vi "ParseControllerPacket.vi"(8 "error in (no error)":errorcluster, 11 "Hex String":string) -> (0 "error out":errorcluster, 3 "Status":T4, 5 "Parameters":T1)   [LabVIEW 2014]
uses:
  Status.ctl
  Parameters.ctl
  PID Mode.ctl
  InputSimulationMode.ctl
panel:
  out "rest of the binary string":string
  out "Binary String":string
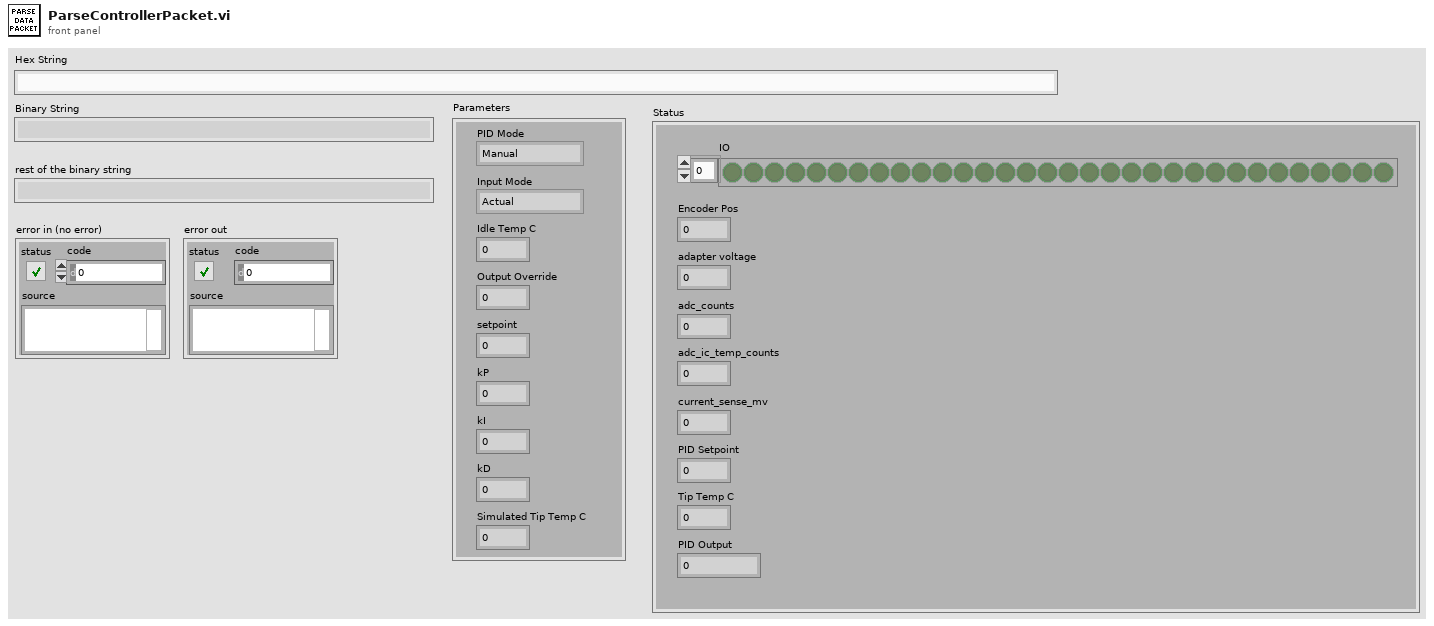
[diagram p1: front panel]
types:
  T1 = typedef "Parameters.ctl" = cluster{"PID Mode":T2, "Input Mode":T3, "Idle Temp C":i16, "Output Override":i16, "setpoint":sgl, "kP":sgl, "kI":sgl, "kD":sgl, "Simulated Tip Temp C":sgl}
  T2 = typedef "PID Mode.ctl" = enum8{"Manual", "Automatic"}
  T3 = typedef "InputSimulationMode.ctl" = enum8{"Actual", "Simulated"}
  T4 = typedef "Status.ctl" = cluster{"IO":bool[], "Encoder Pos":i16, "adapter voltage":i16, "adc_counts":i16, "adc_ic_temp_counts":i16, "current_sense_mv":i16, "PID Setpoint":sgl, "Tip Temp C":sgl, "PID Output":sgl}
  T5 = enum16{"big-endian, network order", "native, host order", "little-endian"}
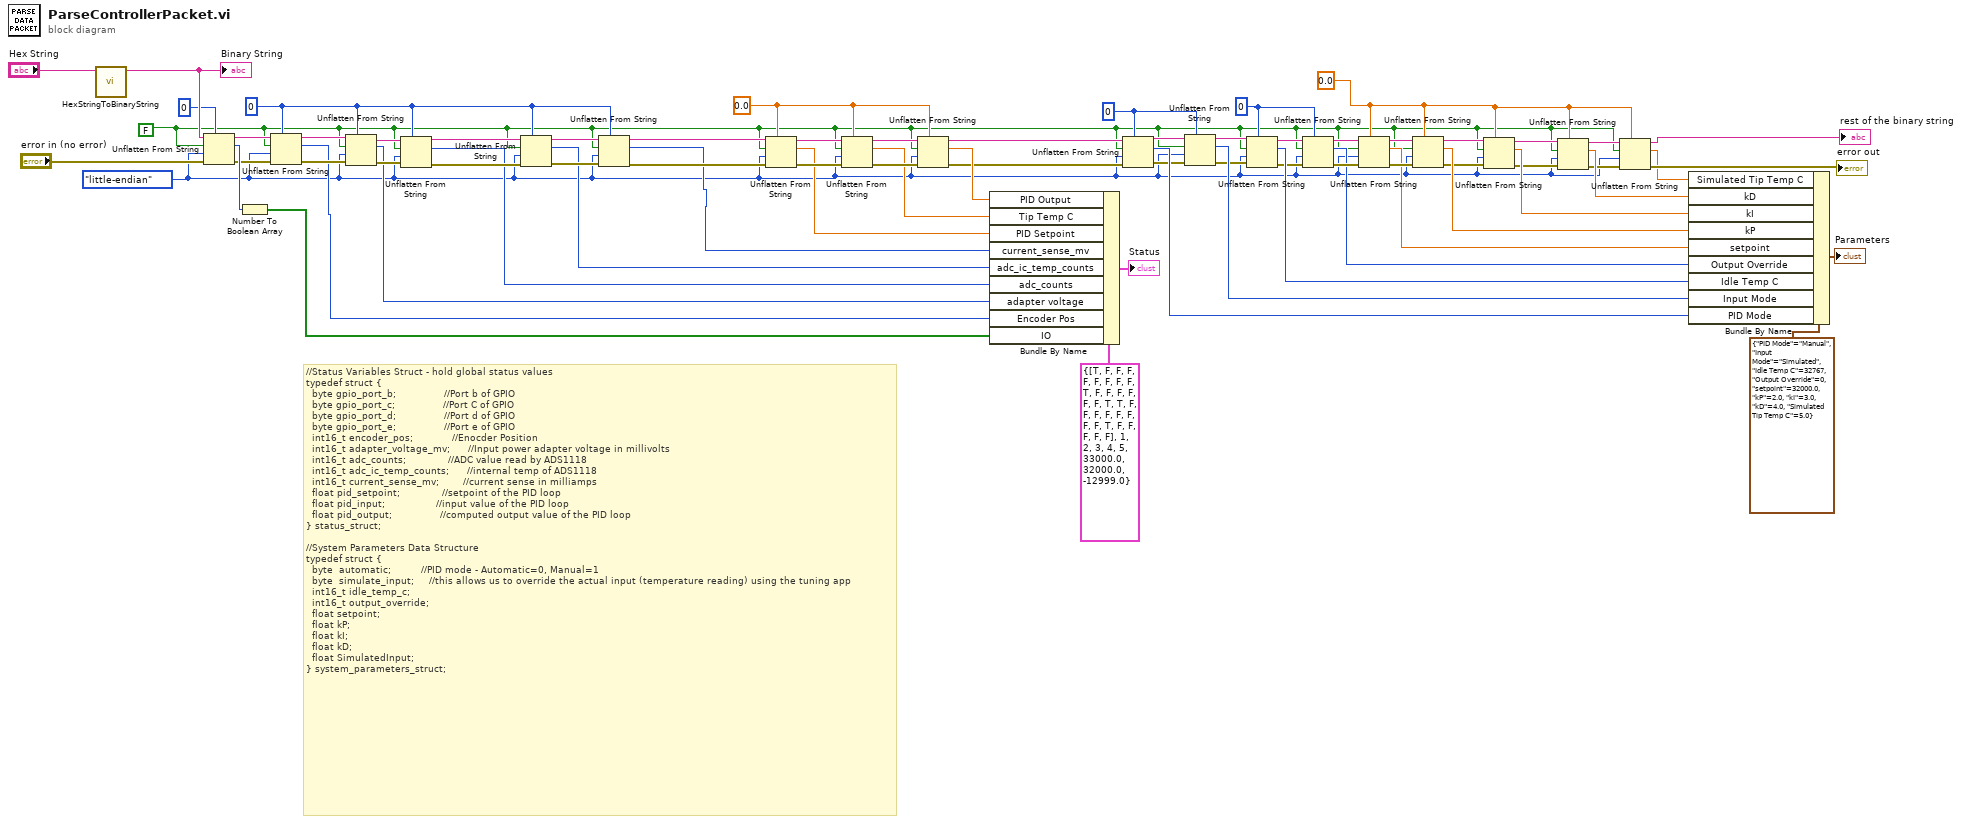
[diagram p0: block diagram]
diagram:
  w4 = sgl 0.0
  w9 = i16 0
  w31 = u8 0
  w49 = sgl 0.0
  w56 = i16 0
  w2 = T5."little-endian" ("byte order (0:big-endian, network order)")
  w3 = FALSE ("data includes array or string size? (T)")
  # "//Status Variables Struct - hold global status values\ntypedef struct {\n  byte gpio_port_b;                //Port b of GPIO\n  byte gpio_port_c;                //Port C of GPIO\n  byte gpio_port_d;                //Port d of GPIO\n  byte gpio_port_e;                //Port e of GPIO\n  int16_t encoder_pos;             //Enocder Position\n  int16_t adapter_voltage_mv;      //Input power adapter voltage in millivolts\n  int16_t adc_counts;              //ADC value read by ADS1118\n  int16_t adc_ic_temp_counts;      //internal temp of ADS1118\n  int16_t current_sense_mv;        //current sense in milliamps\n  float pid_setpoint;              //setpoint of the PID loop\n  float pid_input;                 //input value of the PID loop\n  float pid_output;                //computed output value of the PID loop\n} status_struct;\n\n//System Parameters Data Structure\ntypedef struct {\n  byte  automatic;          //PID mode - Automatic=0, Manual=1\n  byte  simulate_input;     //this allows us to override the actual input (temperature reading) using the tuning app\n  int16_t idle_temp_c;\n  int16_t output_override;\n  float setpoint;\n  float kP;\n  float kI;\n  float kD;\n  float SimulatedInput;\n} system_parameters_struct;"
  n1 = call "HexStringToBinaryString.vi"("Hex String"="Hex String") -> ("Binary String"=w69:string)  [unwired: 10 in]
  "Binary String" <- w69
  n2 = Unflatten From String(type=u32 0, binary string=w69, data includes array or string size? (T)=w3, byte order (0:big-endian, network order)=w2, error in (no error)="error in (no error)") -> (rest of the binary string=w65:string, value=w68:u32, error out=w66:errorcluster)
  n3 = Number To Boolean Array(number=w68) -> (Boolean array=w39:bool[])
  n4 = Unflatten From String(type=w56, binary string=w65, data includes array or string size? (T)=w3, byte order (0:big-endian, network order)=w2, error in (no error)=w66) -> (rest of the binary string=w64:string, value=w40:i16, error out=w63:errorcluster)
  n5 = Unflatten From String(type=w56, binary string=w64, data includes array or string size? (T)=w3, byte order (0:big-endian, network order)=w2, error in (no error)=w63) -> (rest of the binary string=w61:string, value=w41:i16, error out=w62:errorcluster)
  n6 = Unflatten From String(type=w56, binary string=w61, data includes array or string size? (T)=w3, byte order (0:big-endian, network order)=w2, error in (no error)=w62) -> (rest of the binary string=w59:string, value=w42:i16, error out=w60:errorcluster)
  n7 = Unflatten From String(type=w56, binary string=w59, data includes array or string size? (T)=w3, byte order (0:big-endian, network order)=w2, error in (no error)=w60) -> (rest of the binary string=w58:string, value=w43:i16, error out=w57:errorcluster)
  n8 = Unflatten From String(type=w56, binary string=w58, data includes array or string size? (T)=w3, byte order (0:big-endian, network order)=w2, error in (no error)=w57) -> (rest of the binary string=w55:string, value=w44:i16, error out=w54:errorcluster)
  n9 = Unflatten From String(type=w49, binary string=w55, data includes array or string size? (T)=w3, byte order (0:big-endian, network order)=w2, error in (no error)=w54) -> (rest of the binary string=w53:string, value=w45:sgl, error out=w52:errorcluster)
  n10 = Unflatten From String(type=w49, binary string=w53, data includes array or string size? (T)=w3, byte order (0:big-endian, network order)=w2, error in (no error)=w52) -> (rest of the binary string=w51:string, value=w46:sgl, error out=w50:errorcluster)
  n11 = Unflatten From String(type=w49, binary string=w51, data includes array or string size? (T)=w3, byte order (0:big-endian, network order)=w2, error in (no error)=w50) -> (rest of the binary string=w35:string, value=w47:sgl, error out=w36:errorcluster)
  n12 = Bundle By Name(cluster=T4 {"IO"=[TRUE, FALSE, FALSE, FALSE, FALSE, FALSE, FALSE, FALSE, FALSE, TRUE, FALSE, FALSE, FALSE, FALSE, FALSE, FALSE, TRUE, TRUE, FALSE, FALSE, FALSE, FALSE, FALSE, FALSE, FALSE, FALSE, TRUE, FALSE, FALSE, FALSE, FALSE, FALSE], "Encoder Pos"=1, "adapter voltage"=2, "adc_counts"=3, "adc_ic_temp_counts"=4, "current_sense_mv"=5, "PID Setpoint"=33000.0, "Tip Temp C"=32000.0, "PID Output"=-12999.0} ("Status Cluser"), "PID Output"=w47, "Tip Temp C"=w46, "PID Setpoint"=w45, "current_sense_mv"=w44, "adc_ic_temp_counts"=w43, "adc_counts"=w42, "adapter voltage"=w41, "Encoder Pos"=w40, "IO"=w39) -> (→"Status":T4)
  n13 = Unflatten From String(type=w31, binary string=w35, data includes array or string size? (T)=w3, byte order (0:big-endian, network order)=w2, error in (no error)=w36) -> (rest of the binary string=w30:string, value=w33:u8, error out=w29:errorcluster)
  n14 = Unflatten From String(type=w31, binary string=w30, data includes array or string size? (T)=w3, byte order (0:big-endian, network order)=w2, error in (no error)=w29) -> (rest of the binary string=w26:string, value=w28:u8, error out=w27:errorcluster)
  n15 = Unflatten From String(type=w9, binary string=w26, data includes array or string size? (T)=w3, byte order (0:big-endian, network order)=w2, error in (no error)=w27) -> (rest of the binary string=w21:string, value=w25:i16, error out=w24:errorcluster)
  n16 = Unflatten From String(type=w9, binary string=w21, data includes array or string size? (T)=w3, byte order (0:big-endian, network order)=w2, error in (no error)=w24) -> (rest of the binary string=w20:string, value=w18:i16, error out=w23:errorcluster)
  n17 = Unflatten From String(type=w4, binary string=w20, data includes array or string size? (T)=w3, byte order (0:big-endian, network order)=w2, error in (no error)=w23) -> (rest of the binary string=w19:string, value=w17:sgl, error out=w22:errorcluster)
  n18 = Unflatten From String(type=w4, binary string=w19, data includes array or string size? (T)=w3, byte order (0:big-endian, network order)=w2, error in (no error)=w22) -> (rest of the binary string=w14:string, value=w16:sgl, error out=w15:errorcluster)
  n19 = Unflatten From String(type=w4, binary string=w14, data includes array or string size? (T)=w3, byte order (0:big-endian, network order)=w2, error in (no error)=w15) -> (rest of the binary string=w11:string, value=w13:sgl, error out=w12:errorcluster)
  n20 = Unflatten From String(type=w4, binary string=w11, data includes array or string size? (T)=w3, byte order (0:big-endian, network order)=w2, error in (no error)=w12) -> (rest of the binary string=w6:string, value=w10:sgl, error out=w8:errorcluster)
  n21 = Unflatten From String(type=w4, binary string=w6, data includes array or string size? (T)=w3, byte order (0:big-endian, network order)=w2, error in (no error)=w8) -> (rest of the binary string=→"rest of the binary string":string, value=w1:sgl, error out=→"error out":errorcluster)
  n22 = Bundle By Name(cluster=T1 {"PID Mode"=enum."Manual", "Input Mode"=enum."Simulated", "Idle Temp C"=32767, "Output Override"=0, "setpoint"=32000.0, "kP"=2.0, "kI"=3.0, "kD"=4.0, "Simulated Tip Temp C"=5.0} ("Status Cluser"), "Simulated Tip Temp C"=w1, "kD"=w10, "kI"=w13, "kP"=w16, "setpoint"=w17, "Output Override"=w18, "Idle Temp C"=w25, "Input Mode"=w28, "PID Mode"=w33) -> (→"Parameters":T1)
